vi "Inficon - Update recipe list.vi"(8 "Error In":errorcluster, 10 "Metal name":string) -> (0 "Error Out":errorcluster)   [LabVIEW 2014]
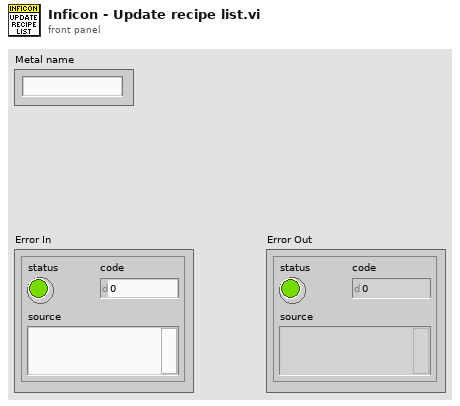
[diagram p1: front panel]
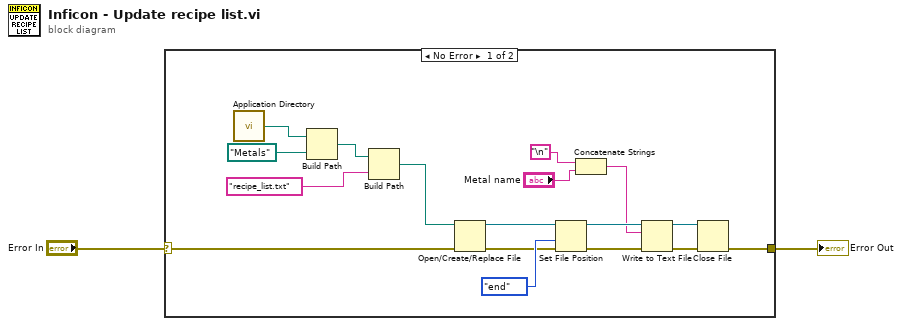
[diagram p0: block diagram]
diagram:
  n1 = case shown="No Error" "Error In" {
    selector: "Error In" -> [w5 w20]
    tunnel: [w6 w20] -> w2
    frame No Error {
      n2 = call <vilib>:"Application Directory.vi"() -> ("Application Directory"=w17:path)
      n3 = Build Path(base path=w17, name or relative path=path "Metals") -> (appended path=w18:path)
      n4 = Build Path(base path=w18, name or relative path="recipe_list.txt" ("string")) -> (appended path=w15:path)
      n5 = Open/Create/Replace File(file path (use dialog)=w15, error in=w5) -> (refnum out=w13:refnum<file>, error out=w10:errorcluster)  [unwired: 4 in, 1 out]
      n6 = Set File Position(refnum=w13, from (0:start)=enum16{"start", "end", "current"}."end", error in=w10) -> (refnum out=w12:refnum<file>, error out=w11:errorcluster)  [unwired: 1 in]
      n7 = Concatenate Strings("\n", "Metal name") -> (w9:string)
      n8 = Write to Text File(file (use dialog)=w12, text=w9, error in=w11) -> (refnum out=w7:refnum<file>, error out=w8:errorcluster)  [unwired: 1 in, 1 out]
      n9 = Close File(refnum=w7, error in=w8) -> (error out=w6:errorcluster)  [unwired: 1 out]
    }
    frame Error {
    }
  }
  "Error Out" <- w2
